vi "FPGA_count_or_not.vi"(10 "Type Counter":enum16{"Falling Edge", "Rising Edge"}(ring), 11 "Countable":bool) -> (3 "Count or Not?":bool)   [LabVIEW 2024]
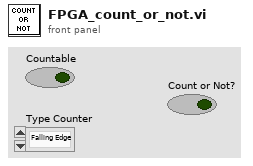
[diagram p1: front panel]
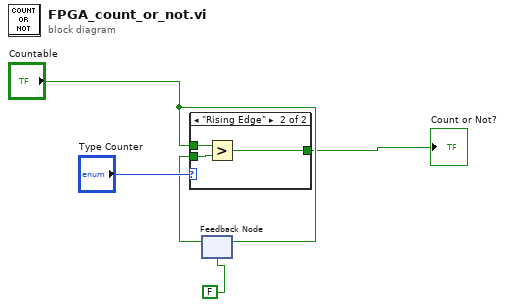
[diagram p0: block diagram]
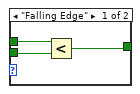
[diagram p2: hidden frame]
diagram:
  n1 = feedback #1(FALSE) -> (w1:bool)
  n2 = case shown="\"Rising Edge\"" "Type Counter" {
    tunnel: w1 -> [w7 w11]
    tunnel: [w6 w10] -> w2
    tunnel: "Countable" -> [w8 w9]
    frame "Falling Edge" {
      n3 = Less?(x=w8, y=w7) -> (x < y?=w6:bool)
    }
    frame "Rising Edge" {
      n4 = Greater?(x=w9, y=w11) -> (0:w10:bool)
    }
  }
  "Count or Not?" <- w2
  n5 = feedback-in #1("Countable") -> ()
